vi "Read_Serial_Pkt.vi"(8 "error in":errorcluster, 11 "VISA resource in":refnum<visa-resource-name>) -> (0 "error out":errorcluster, 1 "Packet OK?":bool, 2 "Data":string, 3 "VISA resource out":refnum<visa-resource-name>)   [LabVIEW 2016]
panel:
  out "Read Count":u32
  out "Pre Sync Rcvd?":bool
  # "remove CRLF from serial config"
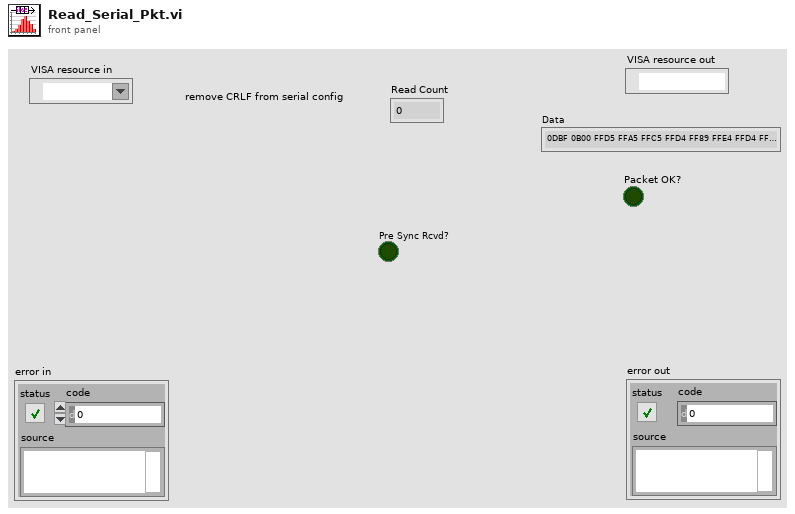
[diagram p1: front panel]
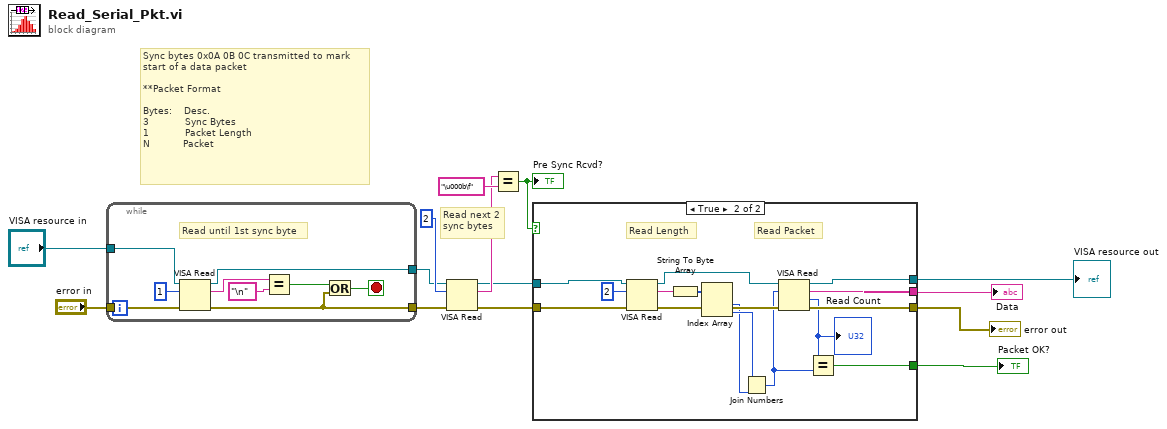
[diagram p0: block diagram]
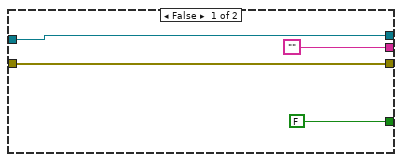
[diagram p2: hidden frame]
diagram:
  # "Sync bytes 0x0A 0B 0C transmitted to mark\nstart of a data packet\n\n**Packet Format\n\nBytes:    Desc.\n3            Sync Bytes\n1            Packet Length\nN           Packet"
  # "Read next 2\nsync bytes"
  n1 = while {
    tunnel: "VISA resource in" -> [w22]
    tunnel: [w17] -> w10
    tunnel: [w16] -> w9
    tunnel: "error in" -> [w15]
    stop <- w19 stop-if-true
    # "Read until 1st sync byte"
    n2 = VISA Read(VISA resource name=w22, byte count=u32 1, error in (no error)=w15) -> (VISA resource name out=w17:refnum<visa-resource-name>, read buffer=w21:string, error out=w16:errorcluster)  [unwired: 1 out]
    n3 = Equal?(x=w21, y="\n") -> (x = y?=w18:bool)
    n4 = Or(x=w18, y=w16) -> (x .or. y?=w19:bool)
  }
  n5 = VISA Read(VISA resource name=w10, byte count=u32 2, error in (no error)=w9) -> (VISA resource name out=w8:refnum<visa-resource-name>, read buffer=w12:string, error out=w7:errorcluster)  [unwired: 1 out]
  n6 = Equal?(x=w12, y="\u000b\f") -> (x = y?=w6:bool)
  "Pre Sync Rcvd?" <- w6
  n7 = case shown="True" w6 {
    tunnel: w8 -> [w27 w41]
    tunnel: w7 -> [w26 w40]
    tunnel: [w27 w34] -> w14
    tunnel: [w26 w35] -> w2
    tunnel: ["" w33] -> w3
    tunnel: [FALSE w31] -> w1
    frame False {
    }
    frame True {
      # "Read Length"
      # "Read Packet"
      n8 = VISA Read(VISA resource name=w41, byte count=u32 2, error in (no error)=w40) -> (VISA resource name out=w39:refnum<visa-resource-name>, read buffer=w37:string, error out=w38:errorcluster)  [unwired: 1 out]
      n9 = String To Byte Array(string=w37) -> (unsigned byte array=w36:u8[])
      n10 = Index Array(array=w36) -> (element #1=w29:u8, element #2=w30:u8)  [unwired: 2 in]
      n11 = Join Numbers(hi=w30, lo=w29) -> ((hi.lo)=w28:u16)
      n12 = VISA Read(VISA resource name=w39, byte count=w28, error in (no error)=w38) -> (VISA resource name out=w34:refnum<visa-resource-name>, read buffer=w33:string, return count=w32:u32, error out=w35:errorcluster)
      "Read Count" <- w32
      n13 = Equal?(x=w32, y=w28) -> (x = y?=w31:bool)
    }
  }
  "error out" <- w2
  "Data" <- w3
  "VISA resource out" <- w14
  "Packet OK?" <- w1
